vi "t-flip-flop.vi"() -> ()   [LabVIEW 2024]
panel:
  out "!Q":bool
  out "Q":bool
  in  "T":bool
  in  "CLK":bool
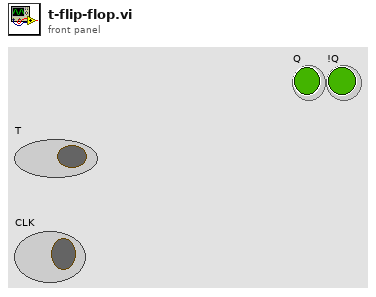
[diagram p1: front panel]
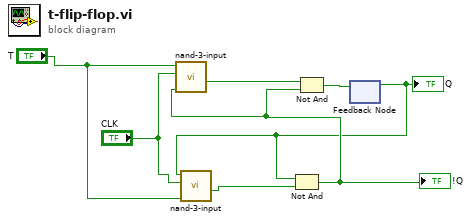
[diagram p0: block diagram]
diagram:
  n1 = feedback #1() -> (w1:bool)  [unwired: 1 in]
  "Q" <- w1
  n2 = call "nand-3-input.vi"("z"="T", "y"="CLK", "x"=w1) -> ("NAND"=w5:bool)  [unwired: 8 in]
  n3 = Not And(1:w5, 2:w1) -> (0:w2:bool)
  "!Q" <- w2
  n4 = call "nand-3-input.vi"("z"=w2, "y"="CLK", "x"="T") -> ("NAND"=w4:bool)  [unwired: 8 in]
  n5 = Not And(1:w2, 2:w4) -> (0:w3:bool)
  n6 = feedback-in #1(w3) -> ()
